vi "Solenoids.vi"() -> ()   [LabVIEW 2016]
panel:
  out "Current State":string
  out "Safe":bool
  out "Filling Out":bool
  out "Aborted":bool
  out "Fill Arm Out":bool
  out "Fire Arm Out":bool
  in  "Filling":bool
  in  "Sensor Warning":bool
  in  "Sensor Data":dbl[](array[numeric])
  in  "Pressurize Command":bool
  in  "Timing Threshold 2":dbl
  in  "Timing Threshold 1":dbl
  in  "PT-1:2E Threshold":dbl
  in  "PT-1:2E":dbl
  in  "Abort Command":bool
  in  "PT-1F Threshold":dbl
  in  "PT-1F":dbl
  in  "PT-1P":dbl
  in  "Fire command":bool
  in  "Fire Arm":bool
  in  "Fill command":bool
  out "Current State":string
  in  "Fill Arm":bool
  out "Spark Plug":bool
  out "Fuel Pump":bool
  out "Firing":bool
  out "Valves":bool[](array[boolean])
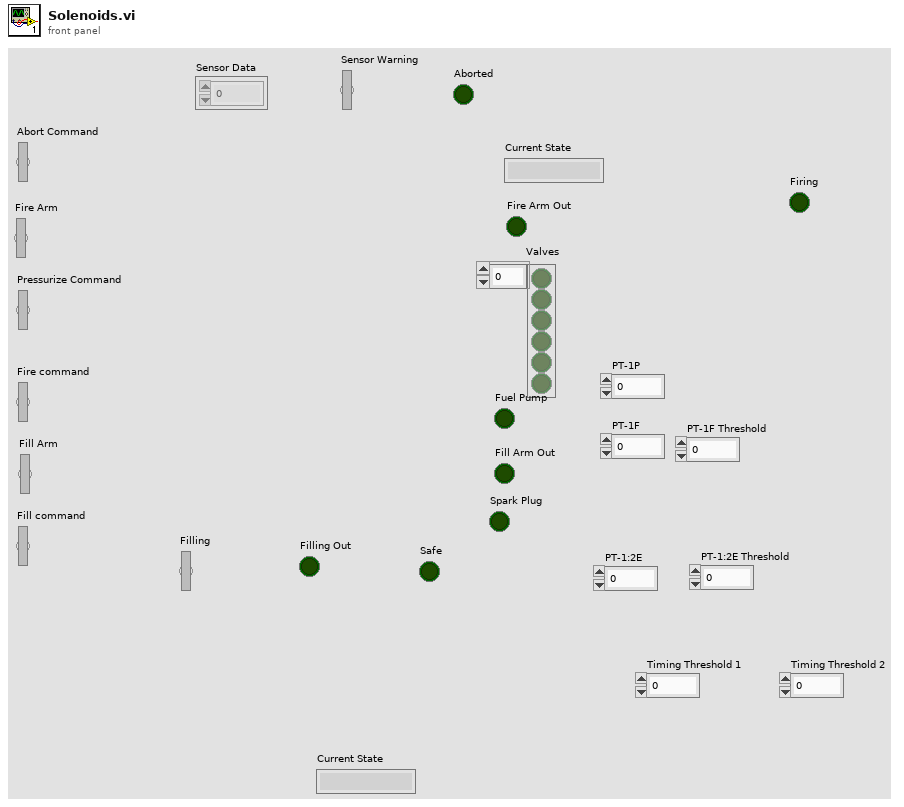
[diagram p1: front panel]
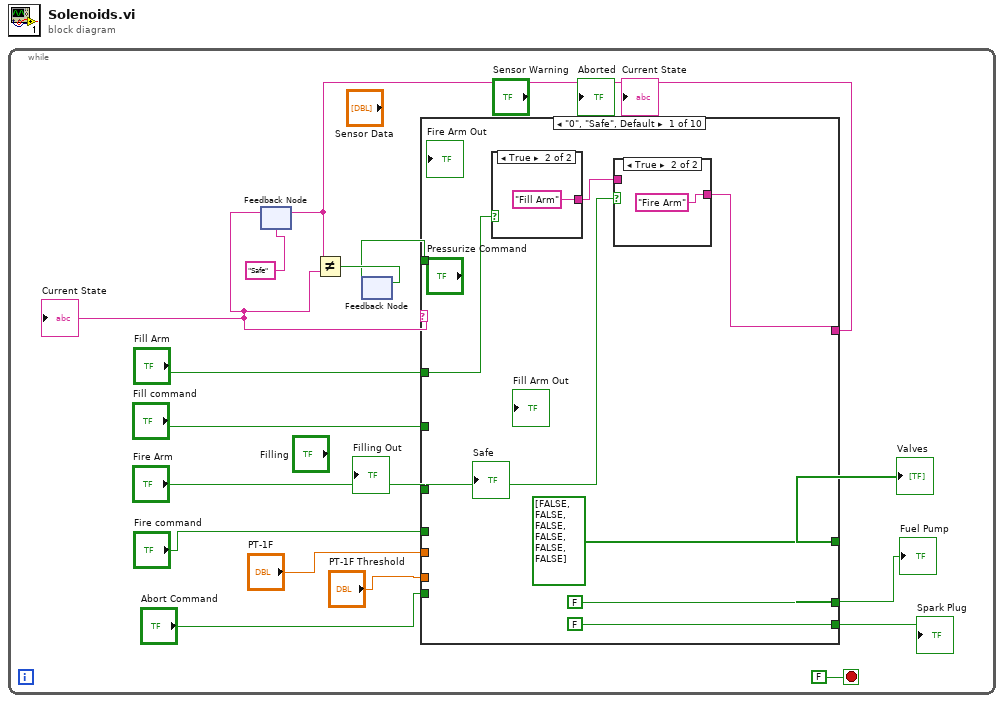
[diagram p0: block diagram]
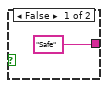
[diagram p3: hidden frame]
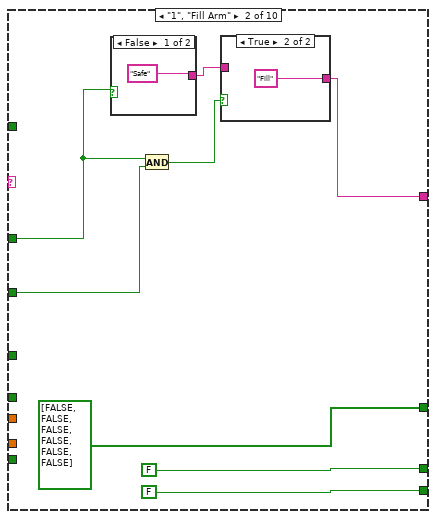
[diagram p4: hidden frame]
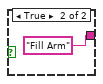
[diagram p6: hidden frame]
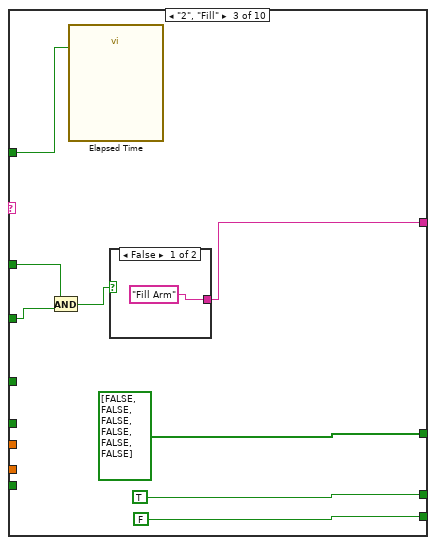
[diagram p7: hidden frame]
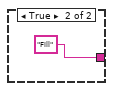
[diagram p8: hidden frame]
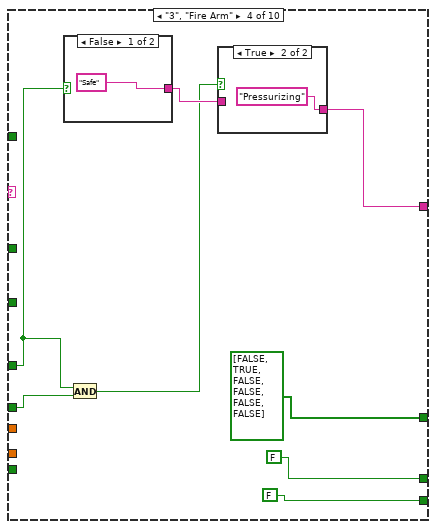
[diagram p9: hidden frame]
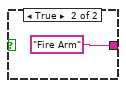
[diagram p11: hidden frame]
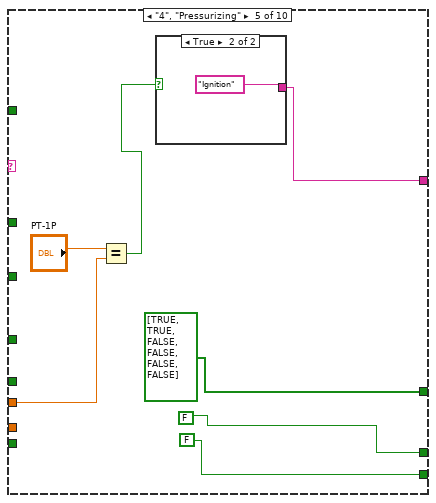
[diagram p12: hidden frame]
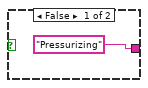
[diagram p13: hidden frame]
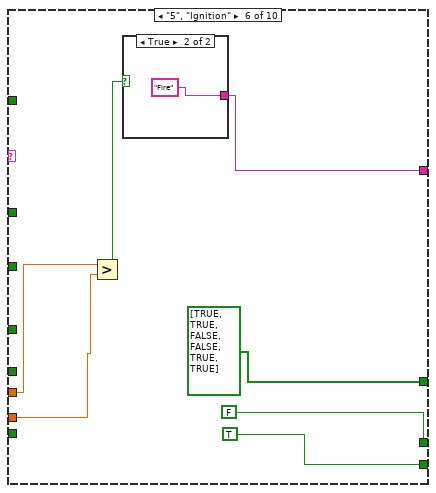
[diagram p14: hidden frame]
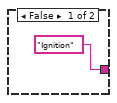
[diagram p15: hidden frame]
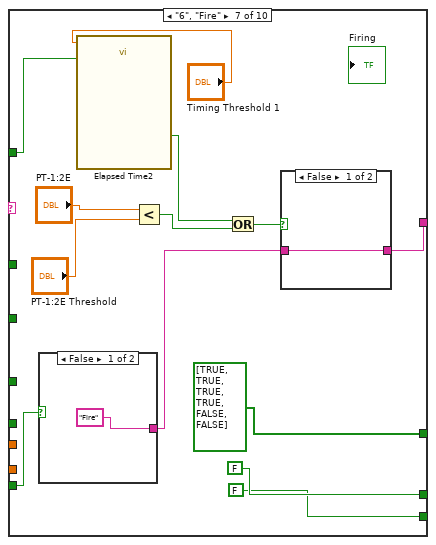
[diagram p16: hidden frame]
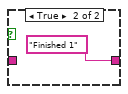
[diagram p17: hidden frame]
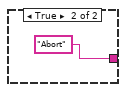
[diagram p18: hidden frame]
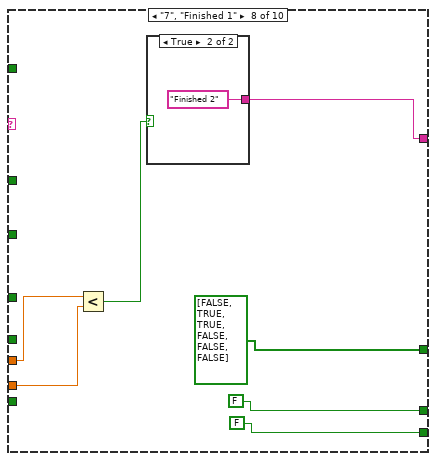
[diagram p19: hidden frame]
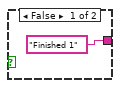
[diagram p20: hidden frame]
diagram:
  n1 = while {
    stop <- FALSE stop-if-true
    n2 = feedback #1("Safe") -> (w10:string)
    "Current State" <- w10
    n3 = feedback #2() -> (w12:bool)  [unwired: 1 in]
    n4 = case shown="\"0\", \"Safe\", Default" w10 {
      tunnel: [w18 w31 w40 w55 w63 w74 w83 w101 w111 w119] -> w8
      tunnel: [bool[] [FALSE, FALSE, FALSE, FALSE, FALSE, FALSE] bool[] [FALSE, FALSE, FALSE, FALSE, FALSE, FALSE] bool[] [FALSE, FALSE, FALSE, FALSE, FALSE, FALSE] bool[] [FALSE, TRUE, FALSE, FALSE, FALSE, FALSE] bool[] [TRUE, TRUE, FALSE, FALSE, FALSE, FALSE] bool[] [TRUE, TRUE, FALSE, FALSE, TRUE, TRUE] bool[] [TRUE, TRUE, TRUE, TRUE, FALSE, FALSE] bool[] [FALSE, TRUE, TRUE, FALSE, FALSE, FALSE] bool[] [FALSE, TRUE, FALSE, FALSE, FALSE, FALSE] bool[] [FALSE, TRUE, FALSE, FALSE, FALSE, FALSE]] -> w6
      tunnel: [FALSE FALSE TRUE FALSE FALSE FALSE FALSE FALSE FALSE FALSE] -> w7
      tunnel: [FALSE FALSE FALSE FALSE FALSE TRUE FALSE FALSE FALSE FALSE] -> w15
      tunnel: "Fill Arm" -> [w20 w28 w43 _ _ _ _ _ _ _]
      tunnel: w12 -> [_ _ w44 _ _ _ w88 _ w112 _]
      tunnel: "Fill command" -> [_ w29 w42 _ _ _ _ _ _ _]
      tunnel: "Fire Arm" -> [w17 _ _ w57 _ _ _ _ _ _]
      tunnel: "Fire command" -> [_ _ _ w56 _ _ _ _ _ _]
      tunnel: "PT-1F" -> [_ _ _ _ w62 w73 _ w103 _ _]
      tunnel: "Abort Command" -> [_ _ _ _ _ _ w89 _ _ w118]
      tunnel: "PT-1F Threshold" -> [_ _ _ _ _ w71 _ w102 _ _]
      frame "0", "Safe", Default {
        n5 = case shown="True" w20 {
          tunnel: ["Safe" "Fill Arm"] -> w19
          frame False {
          }
          frame True {
          }
        }
        n6 = case shown="True" w17 {
          tunnel: [w24 "Fire Arm"] -> w18
          tunnel: w19 -> [w24 _]
          frame False {
          }
          frame True {
          }
        }
      }
      frame "1", "Fill Arm" {
        n7 = case shown="False" w28 {
          tunnel: ["Safe" "Fill Arm"] -> w32
          frame False {
          }
          frame True {
          }
        }
        n8 = And(x=w28, y=w29) -> (x .and. y?=w30:bool)
        n9 = case shown="True" w30 {
          tunnel: [w36 "Fill"] -> w31
          tunnel: w32 -> [w36 _]
          frame False {
          }
          frame True {
          }
        }
      }
      frame "2", "Fill" {
        n10 = And(x=w43, y=w42) -> (x .and. y?=w41:bool)
        n11 = call "Elapsed Time"("Reset"=w44) -> ()  [unwired: 11 in, 8 out]
        n12 = case shown="False" w41 {
          tunnel: ["Fill Arm" "Fill"] -> w40
          frame False {
          }
          frame True {
          }
        }
      }
      frame "3", "Fire Arm" {
        n13 = case shown="False" w57 {
          tunnel: ["Safe" "Fire Arm"] -> w54
          frame False {
          }
          frame True {
          }
        }
        n14 = And(x=w57, y=w56) -> (x .and. y?=w53:bool)
        n15 = case shown="True" w53 {
          tunnel: [w58 "Pressurizing"] -> w55
          tunnel: w54 -> [w58 _]
          frame False {
          }
          frame True {
          }
        }
      }
      frame "4", "Pressurizing" {
        n16 = Equal?(x="PT-1P", y=w62) -> (x = y?=w64:bool)
        n17 = case shown="True" w64 {
          tunnel: ["Pressurizing" "Ignition"] -> w63
          frame False {
          }
          frame True {
          }
        }
      }
      frame "5", "Ignition" {
        n18 = Greater?(x=w73, y=w71) -> (0:w72:bool)
        n19 = case shown="True" w72 {
          tunnel: ["Ignition" "Fire"] -> w74
          frame False {
          }
          frame True {
          }
        }
      }
      frame "6", "Fire" {
        n20 = case shown="False" w89 {
          tunnel: ["Fire" "Abort"] -> w84
          frame False {
          }
          frame True {
          }
        }
        n21 = call "Elapsed Time2"("Time Target (s)"="Timing Threshold 1", "Reset"=w88) -> ("Time has Elapsed"=w80:bool)  [unwired: 10 in, 7 out]
        n22 = Less?(x="PT-1:2E", y="PT-1:2E Threshold") -> (x < y?=w85:bool)
        n23 = Or(x=w80, y=w85) -> (x .or. y?=w82:bool)
        n24 = case shown="False" w82 {
          tunnel: w84 -> [w93 _]
          tunnel: [w93 "Finished 1"] -> w83
          frame False {
          }
          frame True {
          }
        }
      }
      frame "7", "Finished 1" {
        n25 = Less?(x=w103, y=w102) -> (x < y?=w100:bool)
        n26 = case shown="True" w100 {
          tunnel: ["Finished 1" "Finished 2"] -> w101
          frame False {
          }
          frame True {
          }
        }
      }
      frame "8", "Finished 2" {
        n27 = call "Elapsed Time3"("Time Target (s)"="Timing Threshold 2", "Reset"=w112) -> ("Time has Elapsed"=w106:bool)  [unwired: 10 in, 7 out]
        n28 = case shown="True" w106 {
          tunnel: ["Finished 2" "Safe"] -> w111
          frame False {
          }
          frame True {
          }
        }
      }
      frame "9", "Abort" {
        n29 = case shown="False" w118 {
          tunnel: ["Safe" "Abort"] -> w119
          frame False {
          }
          frame True {
          }
        }
      }
    }
    "Spark Plug" <- w15
    "Fuel Pump" <- w7
    "Valves" <- w6
    n30 = feedback-in #1(w8) -> ()
    n31 = Not Equal?(x=w8, y=w10) -> (x != y?=w13:bool)
    n32 = feedback-in #2(w13) -> ()
  }
